vi "Set_RegData_I32.vi"(8 "error in (no error)":errorcluster, 10 "I32":i32, 11 "Class in":refnum<class "IB_RegData_I32.lvclass">) -> (0 "error out":errorcluster, 3 "Class out":refnum<class "IB_RegData_I32.lvclass">)   [LabVIEW 2020, in "IB_RegData_I32.lvclass"]
uses:
  <vilib>/AppBuilder/IB_Classes/RegData/RegData_I32/IB_RegData_I32.lvclass
  <vilib>/AppBuilder/IB_Classes/RegData/RegData_I32/IB_RegData_I32.lvclass/IB_RegData_I32.ctl
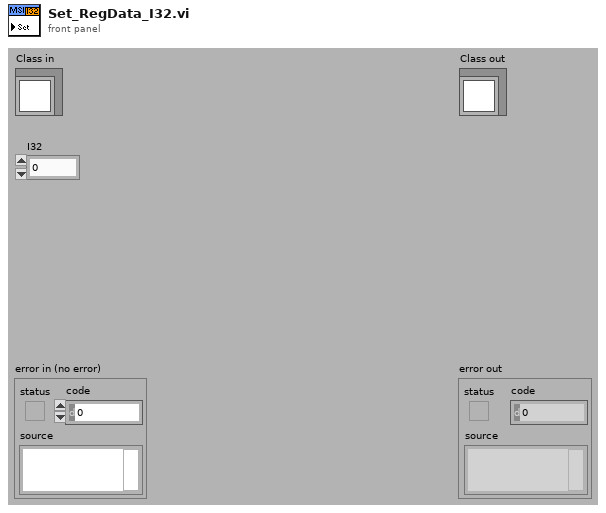
[diagram p1: front panel]
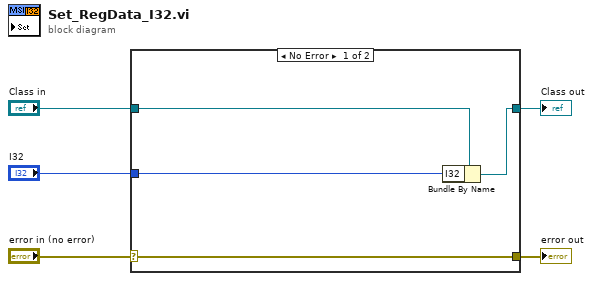
[diagram p0: block diagram]
diagram:
  n1 = case shown="No Error" "error in (no error)" {
    selector: "error in (no error)" -> [w9 w10]
    tunnel: [w9 w10] -> w4
    tunnel: [w7 w11] -> w2
    tunnel: "Class in" -> [w8 w11]
    tunnel: "I32" -> [w6 _]
    frame No Error {
      n2 = Bundle By Name(cluster=w8, "I32"=w6) -> (w7:refnum<class "IB_RegData_I32.lvclass">)
    }
    frame Error {
    }
  }
  "error out" <- w4
  "Class out" <- w2
